vi "test---.vi"() -> ()   [LabVIEW 2019]
panel:
  out "sce-pannel-list out":T1(array[cluster])
  out "sce-pannel-list 2":T2(array[cluster])
  out "sce-pannel-list":T3(array[cluster])
  out "数组 3":cluster{"字符串":string, "数组 2":string[]}[](array[cluster])
  out "数组":string[][](array[string])
  out "模式列表-sorted":T4(array[cluster])
  in  "模式列表 3":T4(array[cluster])=[{"模式"="关|睡眠模式", "sce-pannel-list"=[{"pannel"=[{"ID"=1, "type"="dev", "flag"="", "name"="第三方", "Act"={"Attribute"="", "Action"="open", "Value"=0.0}}, {"ID"=2, "type"="dev", "flag"="", "name"="水电费", "Act"={"Attribute"="", "Action"="close", "Value"=0.0}}, {"ID"=3, "type"="dev", "flag"="", "name"="二", "Act"={"Attribute"="", "Action"="open", "Value"=0.0}}], "pannel-id"=1.0}, {"pannel"=[{"ID"=1, "type"="dev", "flag"="", "name"="而风蛋糕", "Act"={"Attribute"="", "Action"="open", "Value"=0.0}}, {"ID"=2, "type"="dev", "flag"="", "name"="官方", "Act"={"Attribute"="", "Action"="open", "Value"=0.0}}, {"ID"=3, "type"="dev", "flag"="", "name"="俄文", "Act"={"Attribute"="", "Action"="close", "Value"=0.0}}], "pannel-id"=2.0}]}, {"模式"="开|睡眠模式", "sce-pannel-list"=[{"pannel"=[{"ID"=1, "type"="dev", "flag"="", "name"="而风蛋糕", "Act"={"Attribute"="", "Action"="open", "Value"=0.0}}, {"ID"=2, "type"="dev", "flag"="", "name"="官方", "Act"={"Attribute"="", "Action"="open", "Value"=0.0}}, {"ID"=3, "type"="dev", "flag"="", "name"="俄文", "Act"={"Attribute"="", "Action"="close", "Value"=0.0}}], "pannel-id"=2.0}]}, {"模式"="起床模式", "sce-pannel-list"=[{"pannel"=[{"ID"=1, "type"="dev", "flag"="", "name"="而风蛋糕", "Act"={"Attribute"="", "Action"="open", "Value"=0.0}}, {"ID"=2, "type"="dev", "flag"="", "name"="官方", "Act"={"Attribute"="", "Action"="open", "Value"=0.0}}, {"ID"=3, "type"="dev", "flag"="", "name"="俄文", "Act"={"Attribute"="", "Action"="close", "Value"=0.0}}], "pannel-id"=2.0}]}] {"sce-pannel-list"."pannel"."ID" format="%02x"}
  in  "模式列表 4":T4(array[cluster]) {"sce-pannel-list"."pannel"."ID" format="%02x"}
  in  "模式列表 2":T4(array[cluster]) {"sce-pannel-list"."pannel"."ID" format="%02x"}
  in  "模式列表":T4(array[cluster]) {"sce-pannel-list"."pannel"."ID" format="%02x"}
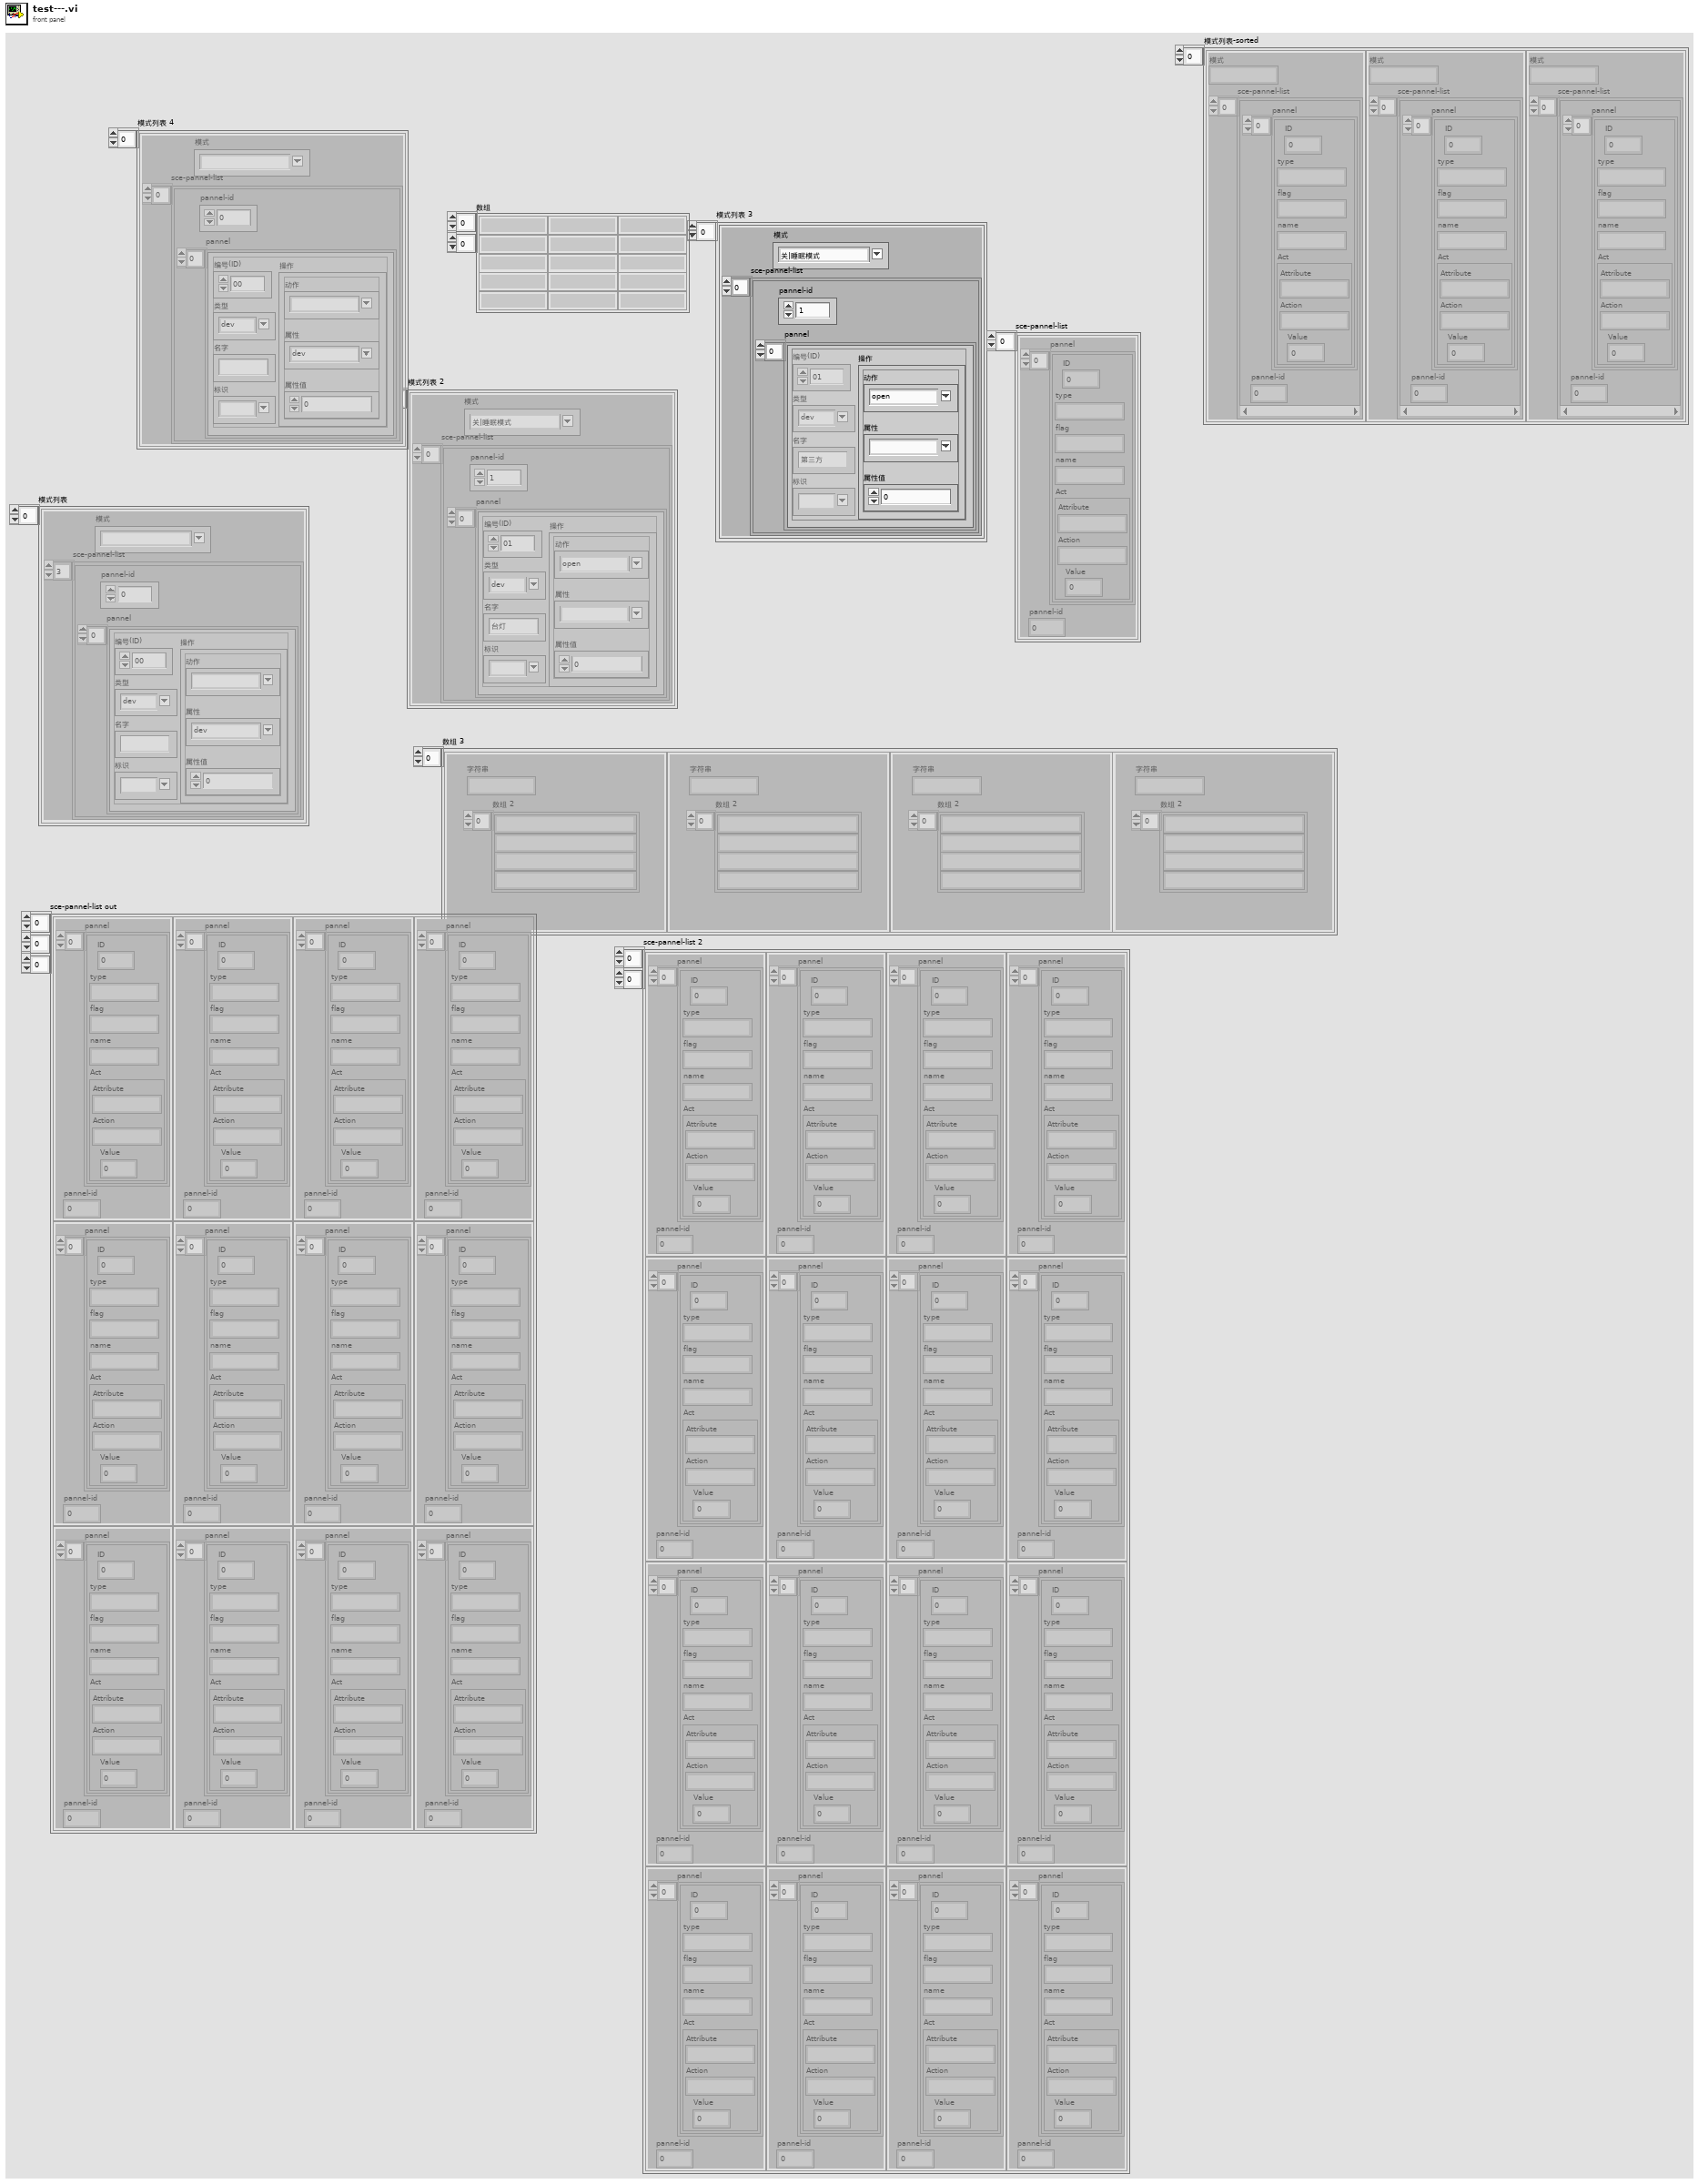
[diagram p1: front panel]
types:
  T1 = cluster{"pannel":cluster{"ID":u8, "type":string, "flag":string, "name":string, "Act":cluster{"Attribute":string, "Action":string, "Value":dbl}}[], "pannel-id":dbl}[][][]
  T2 = cluster{"pannel":cluster{"ID":u8, "type":string, "flag":string, "name":string, "Act":cluster{"Attribute":string, "Action":string, "Value":dbl}}[], "pannel-id":dbl}[][]
  T3 = cluster{"pannel":cluster{"ID":u8, "type":string, "flag":string, "name":string, "Act":cluster{"Attribute":string, "Action":string, "Value":dbl}}[], "pannel-id":dbl}[]
  T4 = cluster{"模式":string, "sce-pannel-list":cluster{"pannel":cluster{"ID":u8, "type":string, "flag":string, "name":string, "Act":cluster{"Attribute":string, "Action":string, "Value":dbl}}[], "pannel-id":dbl}[]}[]
  T5 = cluster{"模式":string, "sce-pannel-list":cluster{"pannel":cluster{"ID":u8, "type":string, "flag":string, "name":string, "Act":cluster{"Attribute":string, "Action":string, "Value":dbl}}[], "pannel-id":dbl}[]}
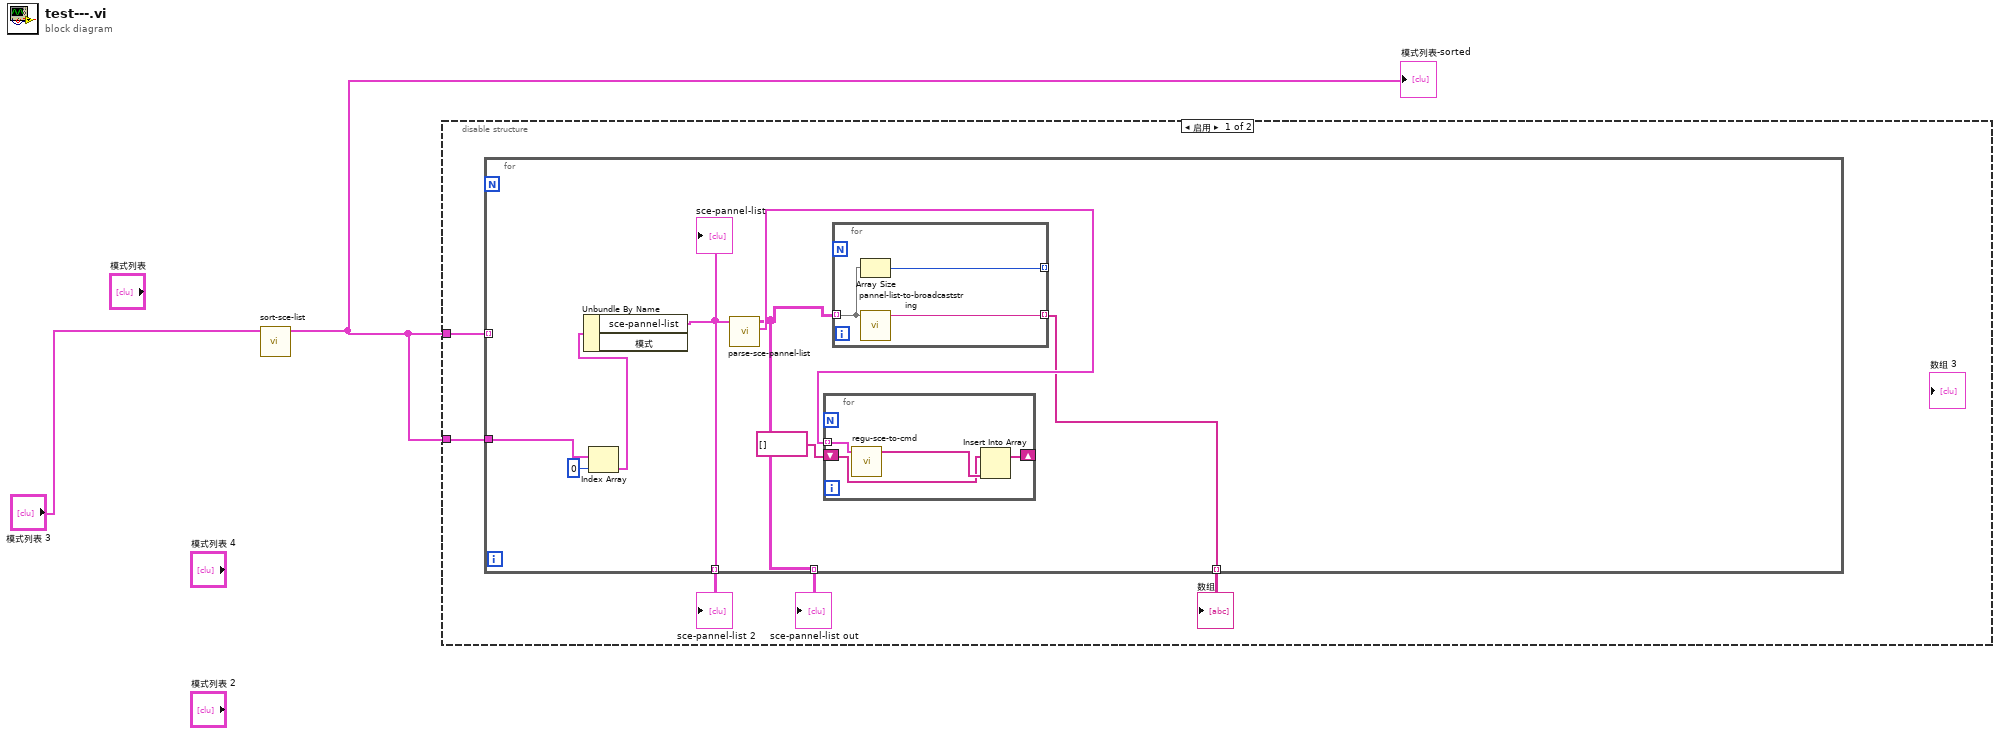
[diagram p0: block diagram]
diagram:
  n1 = call "sort-sce-list.vi"("模式列表"="模式列表 3") -> ("模式列表-sorted"=w1:T4)  [unwired: 10 in]
  "模式列表-sorted" <- w1
  n2 = disable-structure shown="启用" {
    disable-tunnel: w1 -> [w7 _]
    disable-tunnel: w1 -> [w6 _]
    frame Enabled {
      n3 = for {
        tunnel: w7 -> [_] mode=indexing
        tunnel: w6 -> [w14]
        tunnel: [w10] -> w5 mode=indexing
        tunnel: [w9] -> w4 mode=indexing
        tunnel: [w8] -> w3 mode=indexing
        n4 = Index Array(array=w14, index=0 ("索引")) -> (element=w12:T5)
        n5 = Unbundle By Name(w12) -> ("sce-pannel-list"=w9:T3)  [unwired: 1 out]
        "sce-pannel-list" <- w9
        n6 = call "parse-sce-pannel-list.vi"("sce-pannel-list"=w9) -> ("sce-regulate-list"=w15:T3, "sce-pannel-list out"=w8:T2)  [unwired: 9 in]
        n7 = for {
          tunnel: w15 -> [w19] mode=indexing
          shift-right: [w17] -> _
          shift-left: string[] [] -> [w16]
          n8 = call "regu-sce-to-cmd.vi"("regulate-pannel"=w19) -> ("regulate-cmd"=w18:string[])  [unwired: 10 in]
          n9 = Insert Into Array(array=w16, new element=w18) -> (w17:string[])  [unwired: 1 in]
        }
        n10 = for {
          tunnel: w8 -> [w21] mode=indexing
          tunnel: [w22] -> w10 mode=indexing
          tunnel: [w20] -> _ mode=indexing
          n11 = Array Size(array=w21) -> (size(s)=w20:i32)
          n12 = call "pannel-list-to-broadcaststring.vi"("sce-pannel-list"=w21) -> ("sce-pannel-list-cmd"=w22:string)  [unwired: 10 in]
        }
      }
      "数组" <- w5
      "sce-pannel-list 2" <- w4
      "sce-pannel-list out" <- w3
    }
    frame Disabled {
    }
  }
